vi "Create channel list.vi"(11 "Data":T1={"Record heater"=FALSE, "A"=FALSE, "B"=FALSE, "Record RAW"=FALSE, "Set point"=0.0, "Set Heater Range"=enum."0 (Off)", "Approach"=enum."Instant", "Ramp rate, K/min"=1.0, "C"=FALSE, "D"=FALSE}) -> (3 "Array":string[](array[string]))   [LabVIEW 2015]
uses:
  LakeShore340 Front Panel Data.ctl
  LakeShore340 Heater Ranges.ctl
  Neocera/Neocera Set Point Aproach.ctl
panel:
  # "Temperature Monitor"
  # "Record Channels"
  # "Temperature Control"
  # "1 A/50 Ohm\nsee manual\nfor rest"
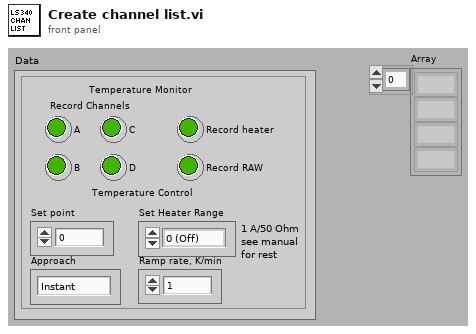
[diagram p1: front panel]
types:
  T1 = typedef "LakeShore340 Front Panel Data.ctl" = cluster{"Record heater":bool, "A":bool, "B":bool, "Record RAW":bool, "Set point":dbl, "Set Heater Range":T2, "Approach":T3, "Ramp rate, K/min":dbl, "C":bool, "D":bool}
  T2 = typedef "LakeShore340 Heater Ranges.ctl" = enum16{"0 (Off)", "1 (5 mW)", "2 (50 mW)", "3 (500 mW)", "4 (5 W)", "5 (50 W)"}
  T3 = typedef "Neocera Set Point Aproach.ctl" = enum16{"Instant", "Ramp"}
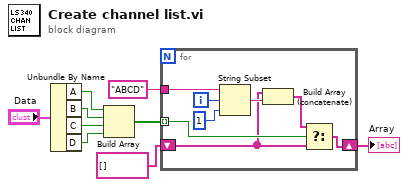
[diagram p0: block diagram]
diagram:
  n1 = Unbundle By Name("Data") -> ("A"=w8:bool, "B"=w7:bool, "C"=w6:bool, "D"=w5:bool)
  n2 = Build Array(w8, w7, w6, w5) -> (w3:bool[])
  n3 = for {
    tunnel: "ABCD" -> [w17]
    tunnel: w3 -> [w13] mode=indexing
    shift-right: [w10] -> w1
    shift-left: string[] [] -> [w11]
    i -> [w16]
    n4 = String Subset(string=w17, offset (0)=w16, length (rest)=1 ("length (rest)")) -> (substring=w15:string)
    n5 = Build Array (concatenate)(w11, w15) -> (w12:string[])
    n6 = Select(t=w12, s=w13, f=w11) -> (s? t:f=w10:string[])
  }
  "Array" <- w1
